vi "Main_Module.vi"(0 "Temperature_Thresholds":T3={"High_Limit(’C)"=70.0, "Low_Limit(’C)"=50.0} caption="Temperature Thresholds", 5 "Start/Stop":T4=TRUE, 11 "Error_In":errorcluster) -> (4 "Alert":T2={"High_Limit_Alert"=TRUE, "Low_Limit_Alert"=FALSE}, 6 "Waveform_Chart":dbl(graph) caption="Chart", 8 "Analysis_Graph":dbl[](graph) caption="Graph", 10 "Analysis_Data":T1={"Maximum_Temperature(’C)"=89.94504794081782, "Minimum_Temperature(’C)"=0.0} caption="Analysis Data", 15 "Error_Out":errorcluster)   [LabVIEW 2021]
uses:
  Controls/Alert.ctl
  Controls/Analysis_Data.ctl
  Controls/Temperature_Thresholds.ctl
  Controls/Start-Stop.ctl
panel:
  # "Temperature Monitor"
  # "Acquisition"
  # "Analysis"
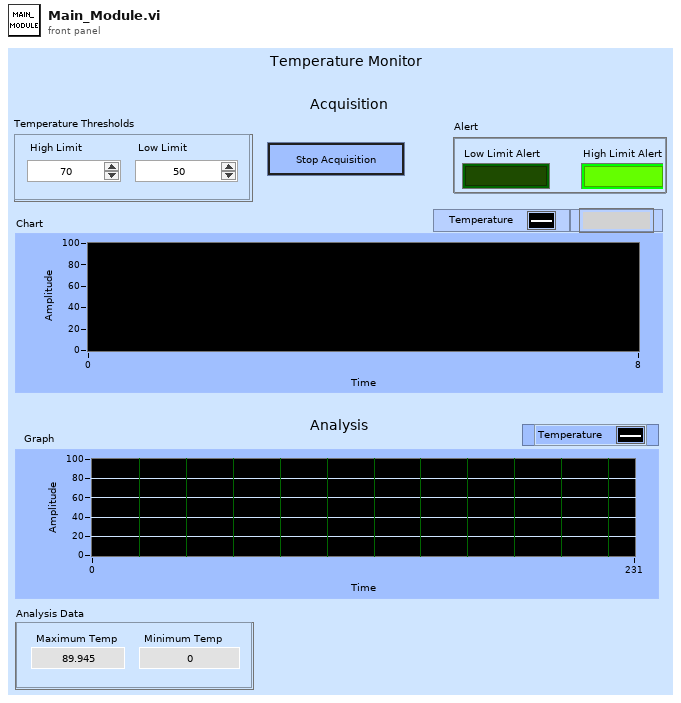
[diagram p1: front panel]
types:
  T1 = typedef "Analysis_Data.ctl" = cluster{"Maximum_Temperature(’C)":dbl, "Minimum_Temperature(’C)":dbl}
  T2 = typedef "Alert.ctl" = cluster{"High_Limit_Alert":bool, "Low_Limit_Alert":bool}
  T3 = typedef "Temperature_Thresholds.ctl" = cluster{"High_Limit(’C)":dbl, "Low_Limit(’C)":dbl}
  T4 = typedef "Start-Stop.ctl" = bool
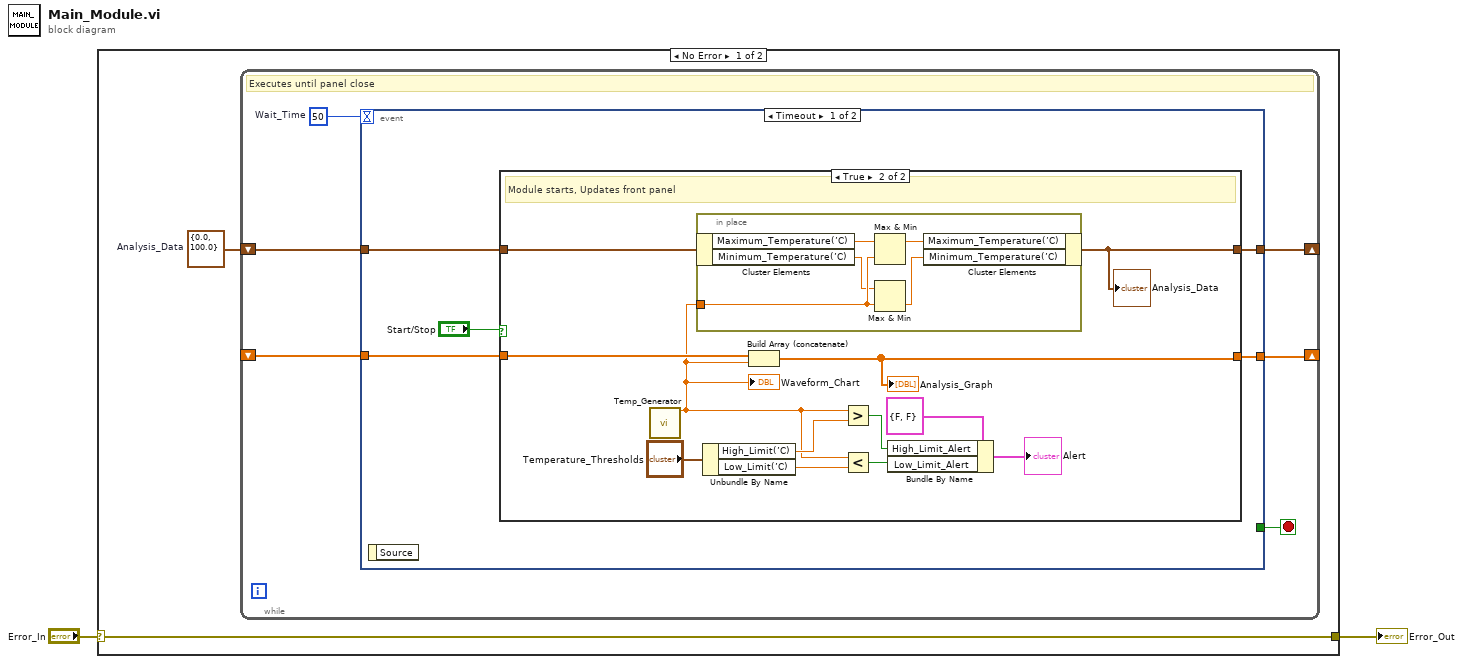
[diagram p0: block diagram]
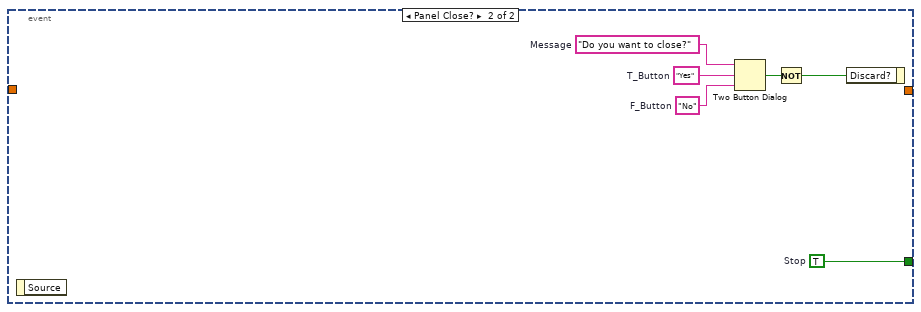
[diagram p3: hidden frame]
diagram:
  n1 = case shown="No Error" "Error_In" {
    selector: "Error_In" -> [w3 w41]
    tunnel: [w3 w41] -> w1
    frame No Error {
      w4 = T1 {"Maximum_Temperature(’C)"=0.0, "Minimum_Temperature(’C)"=100.0}  # Analysis_Data
      n2 = while {
        shift-right: [w7] -> _
        shift-left: _ -> [w8]
        shift-right: [w5] -> _
        shift-left: w4 -> [w6]
        stop <- w9 stop-if-true
        w10 = 50  # Wait_Time
        # "Executes until panel close"
        n3 = event shown="[0] Timeout" {
          selector: _ -> [_ _]
          dyn-events: _ -> [_ _]
          timeout: w10 -> [_ _]
          tunnel: [_ w35] -> w9
          tunnel: w8 -> [w14 _]
          tunnel: [w13 _] -> w7
          tunnel: w6 -> [w12 _]
          tunnel: [w11 _] -> w5
          event Timeout {
            n4 = event-data() -> ()  [unwired: 1 in, 1 out]
            n5 = case shown="True" "Start/Stop" {
              tunnel: w12 -> [w17 w22]
              tunnel: [w17 w21] -> w11
              tunnel: w14 -> [w16 w20]
              tunnel: [w16 w18] -> w13
              frame False {
                # "Module stops, No Updates"
              }
              frame True {
                # "Module starts, Updates front panel"
                n6 = call "Temp_Generator.vi"() -> ("Temp"=w19:dbl)  [unwired: 15 in]
                "Waveform_Chart" <- w19
                n7 = in-place {
                  in-place-border: w19 -> [w34]
                  n8 = in-place-cluster #1(w22) -> ("Maximum_Temperature(’C)"=w33:dbl, "Minimum_Temperature(’C)"=w32:dbl)
                  n9 = Max & Min(x=w33, y=w34) -> (max(x,y)=w31:dbl)  [unwired: 1 out]
                  n10 = Max & Min(x=w32, y=w34) -> (min(x,y)=w30:dbl)  [unwired: 1 out]
                  n11 = in-place-cluster #1("Maximum_Temperature(’C)"=w31, "Minimum_Temperature(’C)"=w30) -> (w21:T1)
                }
                "Analysis_Data" <- w21
                n12 = Unbundle By Name("Temperature_Thresholds") -> ("High_Limit(’C)"=w28:dbl, "Low_Limit(’C)"=w27:dbl)
                n13 = Build Array (concatenate)(w20, w19) -> (w18:dbl[])
                "Analysis_Graph" <- w18
                n14 = Greater?(x=w19, y=w28) -> (0:w26:bool)
                n15 = Less?(x=w19, y=w27) -> (x < y?=w25:bool)
                n16 = Bundle By Name(cluster=T2 {"High_Limit_Alert"=FALSE, "Low_Limit_Alert"=FALSE} ("Alert"), "High_Limit_Alert"=w26, "Low_Limit_Alert"=w25) -> (→"Alert":T2)
              }
            }
          }
          event Panel Close? {
            w35 = TRUE  # Stop
            w38 = "No"  # F_Button
            w39 = "Yes"  # T_Button
            w40 = "Do you want to close?"  # Message
            n17 = event-data() -> ()  [unwired: 1 in, 1 out]
            n18 = Two Button Dialog(message=w40, 1:w38, 2:w39) -> (T button?=w37:bool)
            n19 = Not(x=w37) -> (.not. x?=w36:bool)
            n20 = event-data("Discard?"=w36) -> ()  [unwired: 1 in, 1 out]
          }
        }
      }
    }
    frame Error {
    }
  }
  "Error_Out" <- w1
